vi "Teleop.vi"(10 "Match Info":T1={"Autonomous Elapsed Seconds"=0.0, "TeleOp Elapsed Seconds"=0.0, "Disabled Elapsed Seconds"=0.0, "Visited Autonomous"=FALSE, "Visited TeleOp"=FALSE, "Visited Disabled"=FALSE, "Autonomous Settings"={"Autonomous Style"=enum."Independent", "VI Refnum"=refnum}}, 11 "Call Context":T2) -> ()   [LabVIEW 2017]
doc: "This VI is called for each enabled TeleOp packet received from the DS. It is typically used to read from joysticks and other inputs and update I/O or setpoints for timed control loops. It should complete and return within 20 milliseconds or risk missing DS packets."
uses:
  <vilib>/Rock Robotics/WPI/DriverStation/WPI_DriverStationDerivedRobotMode.ctl
  <vilib>/Rock Robotics/WPI/DriverStation/WPI_DriverStationMatch Info.ctl
  <vilib>/Rock Robotics/WPI/Relay/WPI_RelayValue.ctl
  <vilib>/Rock Robotics/WPI/Solenoid/WPI_SolenoidValue.ctl
  <vilib>/Rock Robotics/WPI/Utilities/WPI_GetSetVariantRefNum.vi
  <vilib>/Rock Robotics/WPI/RobotDrive/WPI_RobotDriveMecanumDrive_Cartesian.vi
  <vilib>/Rock Robotics/WPI/Solenoid/WPI_SolenoidSetEnum.vi
panel:
  out "Distance":dbl
  out "Magnet sensed 2":bool
  out "Magnet sensed 1":bool
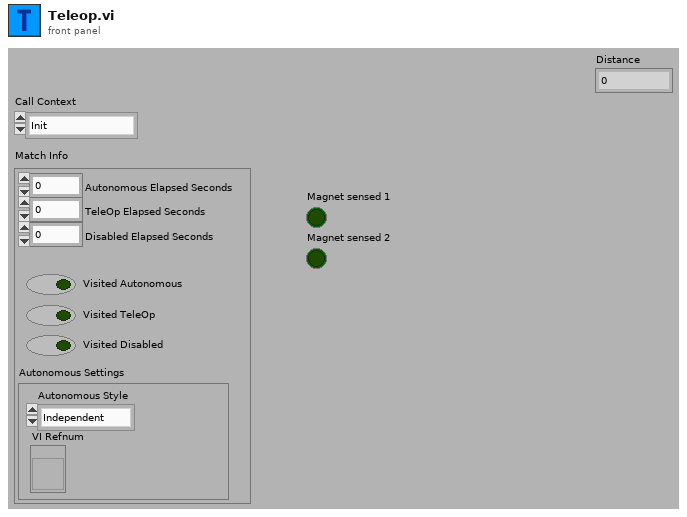
[diagram p1: front panel]
types:
  T1 = typedef "WPI_DriverStationMatch Info.ctl" = cluster{"Autonomous Elapsed Seconds":dbl, "TeleOp Elapsed Seconds":dbl, "Disabled Elapsed Seconds":dbl, "Visited Autonomous":bool, "Visited TeleOp":bool, "Visited Disabled":bool, "Autonomous Settings":cluster{"Autonomous Style":enum16{"Iterative", "Independent"}, "VI Refnum":refnum<vi>}}
  T2 = typedef "WPI_DriverStationDerivedRobotMode.ctl" = enum16{"Init", "Execute", "Stop"}
  T3 = typedef "WPI_SolenoidValue.ctl" = enum16{"Off", "On", "Forward", "Reverse"}
  T4 = typedef "WPI_RelayValue.ctl" = enum16{"Off", "On", "Forward", "Reverse"}
  T5 = typedef "WPI_JoystickDevRef.ctl" = cluster{"Device":T6}
  T6 = typedef "WPI_JoystickDeviceEnum.ctl" = enum16{"USB 0", "USB 1", "USB 2", "USB 3", "USB 4", "USB 5"}
  T7 = typedef "WPI_CompressorDevRef.ctl" = cluster{"DevStatus":errorcluster, "Pneumatics Control Module":u8}
  T8 = typedef "WPI_EncoderDevRef.ctl" = cluster{"DevStatus":errorcluster, "EncoderIndex":T9, "CounterIndex":T10, "DistancePerCount":dbl, "Decoding Type":T11}
  T9 = typedef "FPGA_EncoderIdx.ctl" = enum8{"Enc 0", "Enc 1", "Enc 2", "Enc 3", "Enc 4", "Enc 5", "Enc 6", "Enc 7", "Invalid"}
  T10 = typedef "FPGA_CounterCtrSystemIndex.ctl" = enum8{"Ctr 0", "Ctr 1", "Ctr 2", "Ctr 3", "Ctr 4", "Ctr 5", "Ctr 6", "Ctr 7", "Invalid"}
  T11 = typedef "WPI_EncoderType.ctl" = enum16{"1x", "2x", "4x"}
  T12 = cluster{"Axes[0]":dbl, "Axes[1]":dbl, "Axes[2]":dbl, "Axes[3]":dbl, "Axes[4]":dbl, "Axes[5]":dbl, "Axes[6]":dbl, "Axes[7]":dbl, "Axes[8]":dbl}
  T13 = cluster{"Buttons[0]":bool, "Buttons[1]":bool, "Buttons[2]":bool, "Buttons[3]":bool, "Buttons[4]":bool, "Buttons[5]":bool, "Buttons[6]":bool, "Buttons[7]":bool, "Buttons[8]":bool}
  T14 = typedef "WPI_RobotDriveDevRef.ctl" = cluster{"DevStatus":errorcluster, "Motors[]":T15[], "Square Inputs":bool, "Max Output":dbl}
  T15 = typedef "WPI_MotorControlDeviceRef.ctl" = cluster{"DeviceStatus":errorcluster, "Type":T16, "PWM":cluster{"PWM Channel":T17, "DeadBand":T18}, "CAN":cluster{"Device Number":u8, "SetOutput VI Ref":variant, "GetOutput VI Ref":variant, "Enable VI Ref":variant, "Disable VI Ref":variant, "Data":variant}, "Invert":bool, "DIO PWM":cluster{"PWM \"Enable\" Channel":T17, "DIOChannel":T19, "PWM Rate":dbl}}
  T16 = typedef "WPI_MotorControlType.ctl" = enum16{"PWM", "CAN", "DIO PWM"}
  T17 = typedef "FPGA_DIOPWMChannel.ctl" = enum8{"PWM 0", "PWM 1", "PWM 2", "PWM 3", "PWM 4", "PWM 5", "PWM 6", "PWM 7", "PWM 8", "PWM 9", "PWM MXP 0", "PWM MXP 1", "PWM MXP 2", "PWM MXP 3", "PWM MXP 4", "PWM MXP 5", "PWM MXP 6", "PWM MXP 7", "PWM MXP 8", "PWM MXP 9", "Invalid"}
  T18 = typedef "WPI_PWMDeadband.ctl" = cluster{"Name":string, "maxPositivePwm":i32, "minPositivePwm":i32, "centerPwm":i32, "maxNegativePwm":i32, "minNegativePwm":i32, "angularRange":u16}
  T19 = typedef "FPGA_DIOChannel.ctl" = enum8{"DIO 0", "DIO 1", "DIO 2", "DIO 3", "DIO 4", "DIO 5", "DIO 6", "DIO 7", "DIO 8", "DIO 9", "DIO MXP 0", "DIO MXP 1", "DIO MXP 2", "DIO MXP 3", "DIO MXP 4", "DIO MXP 5", "DIO MXP 6", "DIO MXP 7", "DIO MXP 8", "DIO MXP 9", "DIO MXP 10", "DIO MXP 11", "DIO MXP 12", "DIO MXP 13", "DIO MXP 14", "DIO MXP 15", "SPI Port CS1", "SPI Port CS2", "SPI Port CS3", "SPI Port MISO", "SPI Port MOSI", "Invalid"}
  T20 = typedef "WPI_RelayDevRef.ctl" = cluster{"DevStatus":errorcluster, "Relay Channel":T21, "Relay Direction":T22}
  T21 = typedef "FPGA_DIORelayChannel.ctl" = enum8{"Relay 0", "Relay 1", "Relay 2", "Relay 3", "Invalid"}
  T22 = typedef "WPI_RelayDirection.ctl" = enum16{"Both directions", "Forward only", "Reverse only"}
  T23 = typedef "WPI_SolenoidDevRef.ctl" = cluster{"DevStatus":errorcluster, "Pneumatics Control Module":u8, "Forward Solenoid Channel":T24, "Reverse Solenoid Channel":T24}
  T24 = typedef "WPI_SolenoidChannel.ctl" = enum8{"Solenoid 0", "Solenoid 1", "Solenoid 2", "Solenoid 3", "Solenoid 4", "Solenoid 5", "Solenoid 6", "Solenoid 7", "Invalid"}
  T25 = typedef "WPI_DigitalInputDevRef.ctl" = cluster{"DevStatus":errorcluster, "DIO Channel":T19}
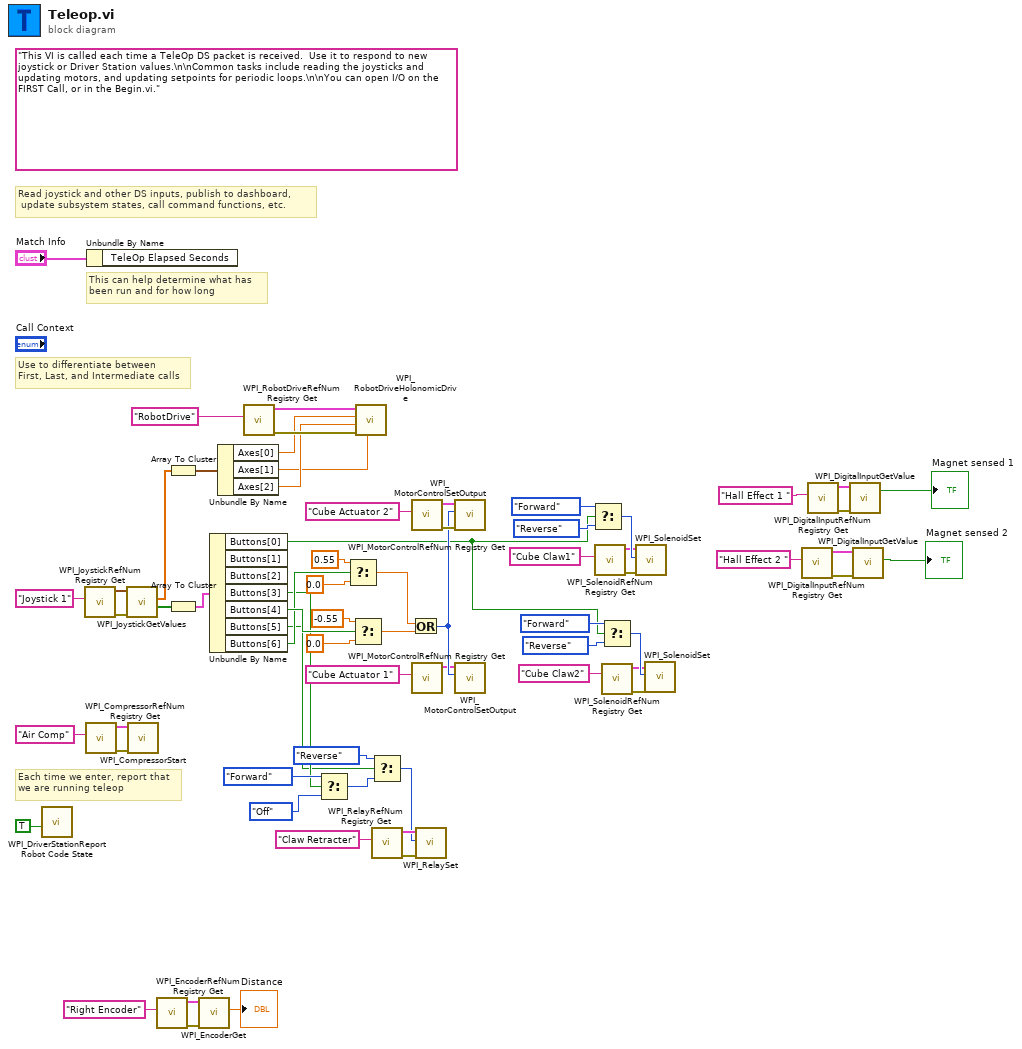
[diagram p0: block diagram]
diagram:
  (unwired) "This VI is called each time a TeleOp DS packet is received.  Use it to respond to new joystick or Driver Station values.\n\nCommon tasks include reading the joysticks and updating motors, and updating setpoints for periodic loops.\n\nYou can open I/O on the FIRST Call, or in the Begin.vi."
  # "Read joystick and other DS inputs, publish to dashboard,\n update subsystem states, call command functions, etc."
  # "Each time we enter, report that\nwe are running teleop"
  # "Use to differentiate between\nFirst, Last, and Intermediate calls"
  # "This can help determine what has\nbeen run and for how long"
  n1 = call <vilib>:"WPI_DriverStationReport Robot Code State.vi"("TeleOp"=TRUE ("Autonomous")) -> ()  [unwired: 10 in, 1 out]
  n2 = call <vilib>:"WPI_JoystickRefNum Registry Get.vi"("refnum name"="Joystick 1") -> ("error out"=w62:errorcluster, "JoystickDevRef"=w61:T5)  [unwired: 9 in]
  n3 = call <vilib>:"WPI_CompressorRefNum Registry Get.vi"("refnum name"="Air Comp") -> ("error out"=w58:errorcluster, "CompressorDevRef"=w57:T7)  [unwired: 9 in]
  n4 = Unbundle By Name("Match Info") -> ()  [unwired: 1 out]
  n5 = call <vilib>:"WPI_JoystickGetValues.vi"("error in (no error)"=w62, "JoystickDevRef"=w61) -> ("Buttons"=w52:bool[], "Axes"=w41:dbl[])  [unwired: 5 in, 3 out]
  n6 = call <vilib>:"WPI_CompressorStart.vi"("error in (no error)"=w58, "CompressorDevRef"=w57) -> ()  [unwired: 8 in, 2 out]
  n7 = call <vilib>:"WPI_EncoderRefNum Registry Get.vi"("refnum name"="Right Encoder") -> ("error out"=w55:errorcluster, "EncoderDevRef"=w56:T8)  [unwired: 9 in]
  n8 = Array To Cluster(array=w41) -> (cluster=w42:T12)
  n9 = Array To Cluster(array=w52) -> (cluster=w51:T13)
  n10 = call <vilib>:"WPI_EncoderGet.vi"("error in (no error)"=w55, "EncoderDevRef"=w56) -> ("Distance"=→"Distance":dbl)  [unwired: 4 in, 5 out]
  n11 = Unbundle By Name(w51) -> ("Buttons[0]"=w7:bool, "Buttons[3]"=w15:bool, "Buttons[4]"=w25:bool, "Buttons[5]"=w14:bool, "Buttons[6]"=w24:bool)  [unwired: 2 out]
  n12 = Unbundle By Name(w42) -> ("Axes[0]"=w40:dbl, "Axes[1]"=w38:dbl, "Axes[2]"=w39:dbl)
  n13 = call <vilib>:"WPI_RobotDriveRefNum Registry Get.vi"("refnum name"="RobotDrive") -> ("error out"=w63:errorcluster, "RobotDriveDevRef"=w64:T14)  [unwired: 9 in]
  n14 = Select(t=WPI_RelayValue."Forward" ("RelayValue"), s=w15, f=WPI_RelayValue."Off" ("RelayValue")) -> (s? t:f=w17:T4)
  n15 = Select(t=0.55, s=w24, f=0.0) -> (s? t:f=w28:dbl)
  n16 = Select(t=-0.55, s=w25, f=0.0) -> (s? t:f=w43:dbl)
  n17 = call-poly <vilib>:"WPI_RobotDriveHolonomicDrive.vi"("Rotation"=w38, "error in (no error)"=w63, "Y"=w39, "X"=w40, "RobotDriveDevRef"=w64) -> ()  [unwired: 4 in, 3 out]
  n18 = Select(t=WPI_RelayValue."Reverse" ("RelayValue"), s=w14, f=w17) -> (s? t:f=w16:T4)
  n19 = call <vilib>:"WPI_RelayRefNum Registry Get.vi"("refnum name"="Claw Retracter") -> ("error out"=w22:errorcluster, "RelayDevRef"=w23:T20)  [unwired: 9 in]
  n20 = Or(x=w28, y=w43) -> (x .or. y?=w34:i32)
  n21 = call <vilib>:"WPI_MotorControlRefNum Registry Get.vi"("refnum name"="Cube Actuator 2") -> ("error out"=w50:errorcluster, "MotorControlDevRef"=w49:T15)  [unwired: 9 in]
  n22 = call <vilib>:"WPI_MotorControlRefNum Registry Get.vi"("refnum name"="Cube Actuator 1") -> ("MotorControlDevRef"=w33:T15)  [unwired: 9 in, 1 out]
  n23 = call <vilib>:"WPI_RelaySet.vi"("error in (no error)"=w22, "RelayValue"=w16, "RelayDevRef"=w23) -> ()  [unwired: 7 in, 2 out]
  n24 = call <vilib>:"WPI_MotorControlSetOutput.vi"("error in (no error)"=w50, "Output"=w34, "MotorControlDevRef"=w49) -> ()  [unwired: 6 in, 3 out]
  n25 = call <vilib>:"WPI_MotorControlSetOutput.vi"("Output"=w34, "MotorControlDevRef"=w33) -> ()  [unwired: 7 in, 3 out]
  n26 = Select(t=WPI_SolenoidValue."Forward" ("Value"), s=w7, f=WPI_SolenoidValue."Reverse" ("Value")) -> (s? t:f=w9:T3)
  n27 = call <vilib>:"WPI_SolenoidRefNum Registry Get.vi"("refnum name"="Cube Claw1") -> ("error out"=w6:errorcluster, "SolenoidDevRef"=w5:T23)  [unwired: 9 in]
  n28 = Select(t=WPI_SolenoidValue."Forward" ("Value"), s=w7, f=WPI_SolenoidValue."Reverse" ("Value")) -> (s? t:f=w8:T3)
  n29 = call <vilib>:"WPI_SolenoidRefNum Registry Get.vi"("refnum name"="Cube Claw2") -> ("error out"=w2:errorcluster, "SolenoidDevRef"=w3:T23)  [unwired: 9 in]
  n30 = call-poly <vilib>:"WPI_SolenoidSet.vi"("error in (no error)"=w6, "Value"=w9, "SolenoidDevRef"=w5) -> ()  [unwired: 7 in, 2 out]
  n31 = call-poly <vilib>:"WPI_SolenoidSet.vi"("error in (no error)"=w2, "Value"=w8, "SolenoidDevRef"=w3) -> ()  [unwired: 7 in, 2 out]
  n32 = call <vilib>:"WPI_DigitalInputRefNum Registry Get.vi"("refnum name"="Hall Effect 2 ") -> ("error out"=w30:errorcluster, "DigitalInputDevRef"=w31:T25)  [unwired: 9 in]
  n33 = call <vilib>:"WPI_DigitalInputRefNum Registry Get.vi"("refnum name"="Hall Effect 1 ") -> ("error out"=w35:errorcluster, "DigitalInputDevRef"=w36:T25)  [unwired: 9 in]
  n34 = call <vilib>:"WPI_DigitalInputGetValue.vi"("error in (no error)"=w35, "DigitalInputDevRef"=w36) -> ("Value"=→"Magnet sensed 1":bool)  [unwired: 7 in, 2 out]
  n35 = call <vilib>:"WPI_DigitalInputGetValue.vi"("error in (no error)"=w30, "DigitalInputDevRef"=w31) -> ("Value"=→"Magnet sensed 2":bool)  [unwired: 7 in, 2 out]
